vi "Get Encoder Angles.vi"() -> (0 "output cluster":T1)   [LabVIEW 2018]
uses:
  Encoder Unpacked Data.ctl
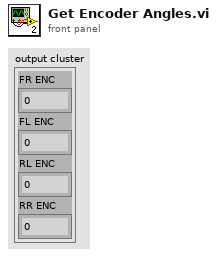
[diagram p1: front panel]
types:
  T1 = typedef "Encoder Unpacked Data.ctl" = cluster{"FR ENC":dbl, "FL ENC":dbl, "RL ENC":dbl, "RR ENC":dbl}
  T2 = typedef "WPI_AnalogChannelDevRef.ctl" = cluster{"DevStatus":errorcluster, "Analog Channel":T3}
  T3 = typedef "FPGA_AIChannel.ctl" = enum8{"AI 0", "AI 1", "AI 2", "AI 3", "AI MXP 0", "AI MXP 1", "AI MXP 2", "AI MXP 3", "Invalid"}
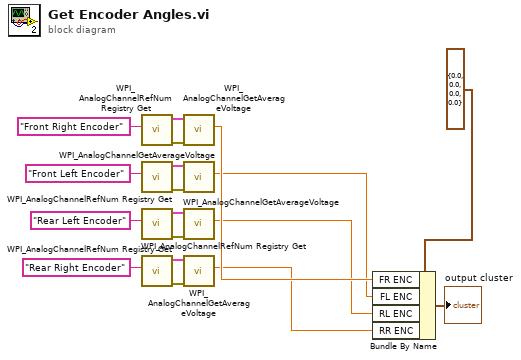
[diagram p0: block diagram]
diagram:
  n1 = call <vilib>:"WPI_AnalogChannelRefNum Registry Get.vi"("refnum name"="Front Right Encoder") -> ("error out"=w15:errorcluster, "AIDeviceRef"=w14:T2)  [unwired: 9 in]
  n2 = call <vilib>:"WPI_AnalogChannelRefNum Registry Get.vi"("refnum name"="Front Left Encoder") -> ("error out"=w12:errorcluster, "AIDeviceRef"=w11:T2)  [unwired: 9 in]
  n3 = call <vilib>:"WPI_AnalogChannelRefNum Registry Get.vi"("refnum name"="Rear Left Encoder") -> ("error out"=w18:errorcluster, "AIDeviceRef"=w17:T2)  [unwired: 9 in]
  n4 = call <vilib>:"WPI_AnalogChannelRefNum Registry Get.vi"("refnum name"="Rear Right Encoder") -> ("error out"=w9:errorcluster, "AIDeviceRef"=w8:T2)  [unwired: 9 in]
  n5 = call <vilib>:"WPI_AnalogChannelGetAverageVoltage.vi"("error in (no error)"=w15, "AIDeviceRef"=w14) -> ("Voltage"=w5:dbl)  [unwired: 7 in, 2 out]
  n6 = call <vilib>:"WPI_AnalogChannelGetAverageVoltage.vi"("error in (no error)"=w12, "AIDeviceRef"=w11) -> ("Voltage"=w4:dbl)  [unwired: 7 in, 2 out]
  n7 = call <vilib>:"WPI_AnalogChannelGetAverageVoltage.vi"("error in (no error)"=w18, "AIDeviceRef"=w17) -> ("Voltage"=w3:dbl)  [unwired: 7 in, 2 out]
  n8 = call <vilib>:"WPI_AnalogChannelGetAverageVoltage.vi"("error in (no error)"=w9, "AIDeviceRef"=w8) -> ("Voltage"=w2:dbl)  [unwired: 7 in, 2 out]
  n9 = Bundle By Name(cluster=T1 {"FR ENC"=0.0, "FL ENC"=0.0, "RL ENC"=0.0, "RR ENC"=0.0}, "FR ENC"=w5, "FL ENC"=w4, "RL ENC"=w3, "RR ENC"=w2) -> (→"output cluster":T1)
